vi "Amplitude and Levels 1 chan.vi"(6 "state settings":T1={"method"=enum."auto select", "histogram size"=256, "histogram method"=enum."mode", "reserved"=1.0} {"reserved" format="%0.2f"}, 8 "error in (no error)":errorcluster, 11 "signal in":waveform(dbl)) -> (0 "error out":errorcluster, 1 "low state level":dbl format="%.2g", 2 "high state level":dbl format="%.2g", 3 "amplitude":dbl format="%.2p")   [LabVIEW 2020, in "NI_MAPro.lvlib"]
doc: "Returns the <B>amplitude</B>, <B>high state level</B>, and <B>low state level</B> of a waveform or an array of waveforms. Wire data to the <B>signal in</B> input to determine the polymorphic instance to use or manually select the instance."
uses:
  NI_MAPro.lvlib
  NI_MABase.lvlib
  <resource>/lvanlys.dll
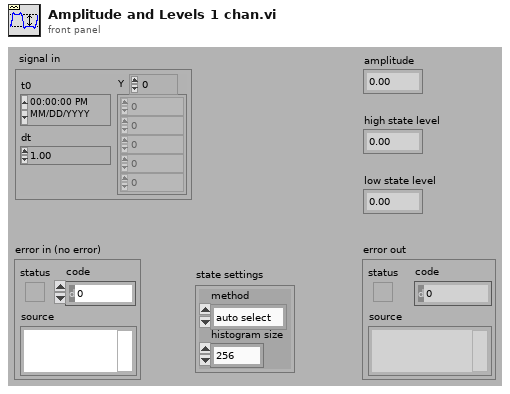
[diagram p1: front panel]
types:
  T1 = cluster{"method":enum32{"histogram", "peak", "auto select"}, "histogram size":i32, "histogram method":enum16{"mode"}, "reserved":dbl}
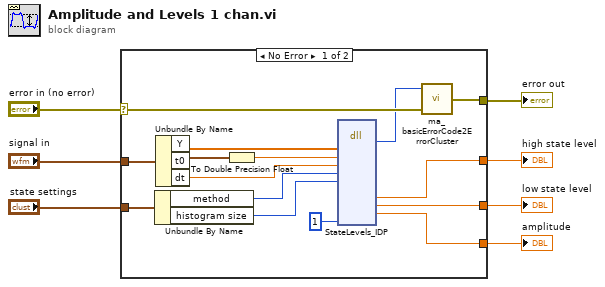
[diagram p0: block diagram]
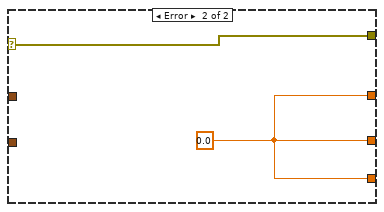
[diagram p2: hidden frame]
diagram:
  n1 = case shown="No Error" "error in (no error)" {
    selector: "error in (no error)" -> [w16 w24]
    tunnel: [w20 w24] -> w1
    tunnel: "signal in" -> [w22 _]
    tunnel: "state settings" -> [w21 _]
    tunnel: [w19 w23] -> w4
    tunnel: [w18 w23] -> w3
    tunnel: [w17 w23] -> w2
    frame No Error {
      n2 = Unbundle By Name(w21) -> ("method"=w12:enum32{"histogram", "peak", "auto select"}, "histogram size"=w11:i32)
      n3 = Unbundle By Name(w22) -> ("Y"=w10:dbl[], "t0"=w13:timestamp, "dt"=w15:dbl)
      n4 = To Double Precision Float(number=w13) -> (double precision float=w14:dbl)
      n5 = dll-call lib="C:/Program Files (x86)/National Instruments/LabVIEW 2020/resource/lvanlys.*" fn="StateLevels_IDP"("xH"=w10, "Xo"=w14, "dx"=w15, "method"=w12, "histoSize"=w11, "newAlgorithm"=1) -> ("return type"=w8:i32, "high"=w19:dbl, "low"=w18:dbl, "amp"=w17:dbl)  [unwired: 10 in, 6 out]
      n6 = call "ma_basicErrorCode2ErrorCluster.vi"("error in (no error)"=w16, "Error Code"=w8) -> ("error out"=w20:errorcluster)  [unwired: 1 in]
    }
    frame Error {
      w23 = 0.0 ("high")
    }
  }
  "amplitude" <- w2
  "low state level" <- w3
  "error out" <- w1
  "high state level" <- w4
